vi "读取CODMn数据波形.vi"() -> ()   [LabVIEW 2016]
uses:
  System.Windows.Forms
  <vilib>/DataGrid for LabVIEW/source/GridColumn/ColumnDefinition.ctl
  <vilib>/DataGrid for LabVIEW/source/GridColumn/ColumnType.ctl
  <vilib>/Utility/miscctls.llb/LVPointTypeDef.ctl
  <vilib>/Waveform/WDTFileIO.llb/Read Waveform from File.vi
  <vilib>/DataGrid for LabVIEW/source/DataGridView/DataGridView.lvclass
  D:/Program Files (x86)/National Instruments/LabVIEW 2016/examples/DataGrid for LabVIEW/DataGrid.lvlib
  <vilib>/DataGrid for LabVIEW/source/Events/CellValueChanged/CellValueChanged.lvclass
  <vilib>/DataGrid for LabVIEW/source/Events/CellClick/CellClick.lvclass
  <vilib>/DataGrid for LabVIEW/source/Events/KeyDown/KeyDown.lvclass
  <vilib>/DataGrid for LabVIEW/source/GridColumn/GridColumn.lvclass
panel:
  in  "进度值":i32
  in  "当前温度曲线":bool
  out "下拉列表":u16(ring)
  in  "Discard?":bool
  in  "查询":bool
  in  "簇":cluster{"数据起始时间":timestamp, "数据终止时间":timestamp}
  in  "当前滴定曲线":bool
  in  "打开波形文件":bool
  in  "关闭":bool
  out "数组":T2(array[cluster]) {"MinWidth" min=2 step=1; "AutoSizeMode" items=["None"=1, "ColumnHeader"=2, "AllCellsExceptHeader"=4, "AllCells"=6, "DisplayedCellsExceptHeader"=8, "DisplayedCells"=10, "Fill"=16]; "FillWeight" min=1 max=100}
  out "Events":string
  in  "# of Rows":i32=15
  in  "ColumnSetup":T3[](array[typedef])=[{"name"="Text", "caption"="Text", "datatype"=enum."string", "Params"="", "AutoSizeMode"=2, "FillWeight"=10.0, "MinWidth"=25, "tooltip"="Text The quick brown fox jumps over the lazy dog"}, {"name"="Details", "caption"="Details", "datatype"=enum."string", "Params"="", "AutoSizeMode"=16, "FillWeight"=100.0, "MinWidth"=150, "tooltip"="Details The quick brown fox jumps over the lazy dog"}, {"name"="Time", "caption"="", "datatype"=enum."timestamp", "Params"="", "AutoSizeMode"=1, "FillWeight"=1.0, "MinWidth"=120, "tooltip"="Time The quick brown fox jumps over the lazy dog"}, {"name"="Selection", "caption"="", "datatype"=enum."combo", "Params"="One|Two|Three", "AutoSizeMode"=6, "FillWeight"=1.0, "MinWidth"=80, "tooltip"="Selection The quick brown fox jumps over the lazy dog"}, {"name"="Function", "caption"="", "datatype"=enum."button", "Params"="", "AutoSizeMode"=6, "FillWeight"=1.0, "MinWidth"=50, "tooltip"="Function The quick brown fox jumps over the lazy dog"}, {"name"="Value", "caption"="", "datatype"=enum."numeric", "Params"="", "AutoSizeMode"=6, "FillWeight"=1.0, "MinWidth"=10, "tooltip"="Value The quick brown fox jumps over the lazy dog"}, {"name"="Active", "caption"="", "datatype"=enum."check", "Params"="", "AutoSizeMode"=6, "FillWeight"=1.0, "MinWidth"=10, "tooltip"=""}, {"name"="Status", "caption"="", "datatype"=enum."image", "Params"="", "AutoSizeMode"=6, "FillWeight"=1.0, "MinWidth"=10, "tooltip"=""}, {"name"="Link", "caption"="", "datatype"=enum."link", "Params"="", "AutoSizeMode"=1, "FillWeight"=100.0, "MinWidth"=50, "tooltip"=""}] {"MinWidth" min=2 step=1; "AutoSizeMode" items=["None"=1, "ColumnHeader"=2, "AllCellsExceptHeader"=4, "AllCells"=6, "DisplayedCellsExceptHeader"=8, "DisplayedCells"=10, "Fill"=16]; "FillWeight" min=1 max=100}
  in  "DataGridView":refnum<k24>(container)
  # "加载中，请稍后......"
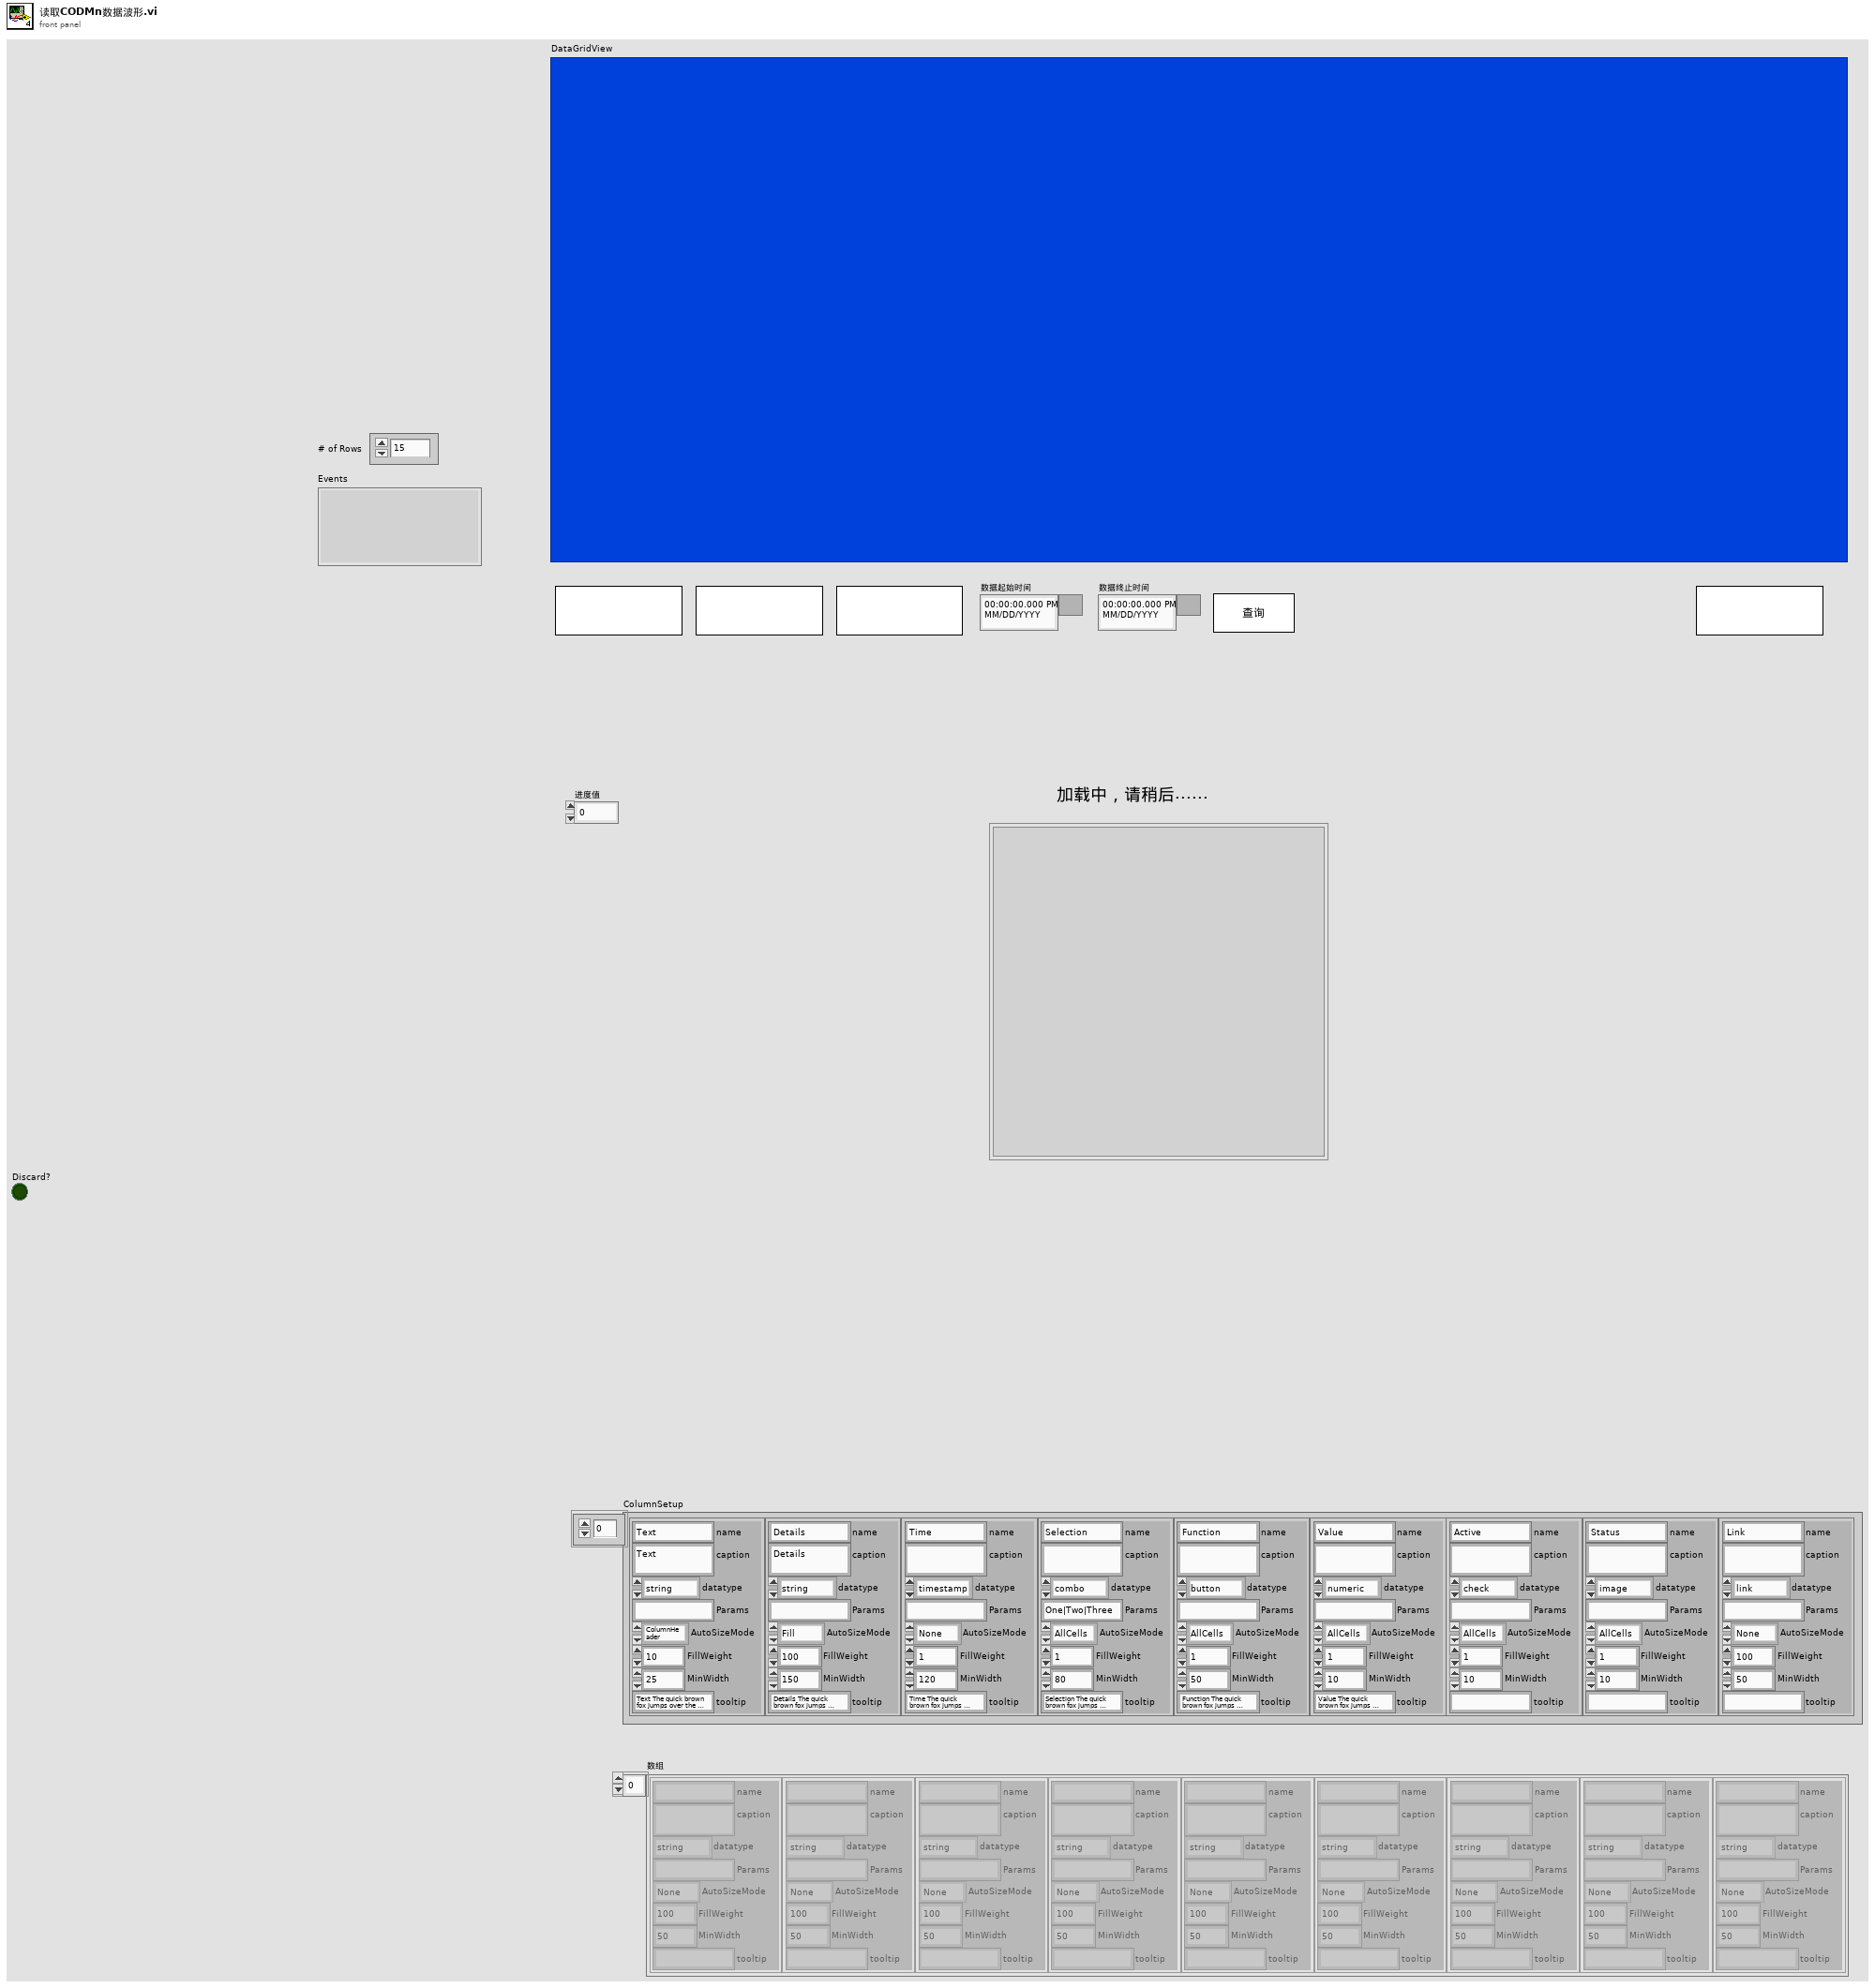
[diagram p1: front panel]
types:
  T1 = typedef "DataGrid.lvlib/GridColumn.lvclass/ColumnType.ctl" = enum16{"string", "image", "check", "numeric", "timestamp", "button", "combo", "link"}
  T2 = cluster{"name":string, "caption":string, "datatype":T1, "Params":string, "AutoSizeMode":i32, "FillWeight":sgl, "MinWidth":u32, "tooltip":string}[]
  T3 = typedef "DataGrid.lvlib/GridColumn.lvclass/ColumnDefinition.ctl" = cluster{"name":string, "caption":string, "datatype":T1, "Params":string, "AutoSizeMode":i32, "FillWeight":sgl, "MinWidth":u32, "tooltip":string}
  T4 = typedef "LVPointTypeDef.ctl" = cluster{"Horizontal":i16, "Vertical":i16}
  T5 = cluster{"Alt":bool, "Control":bool, "KeyCode":i32, "KeyData":i32, "KeyValue":i32, "Modifiers":i32, "Shift":bool}
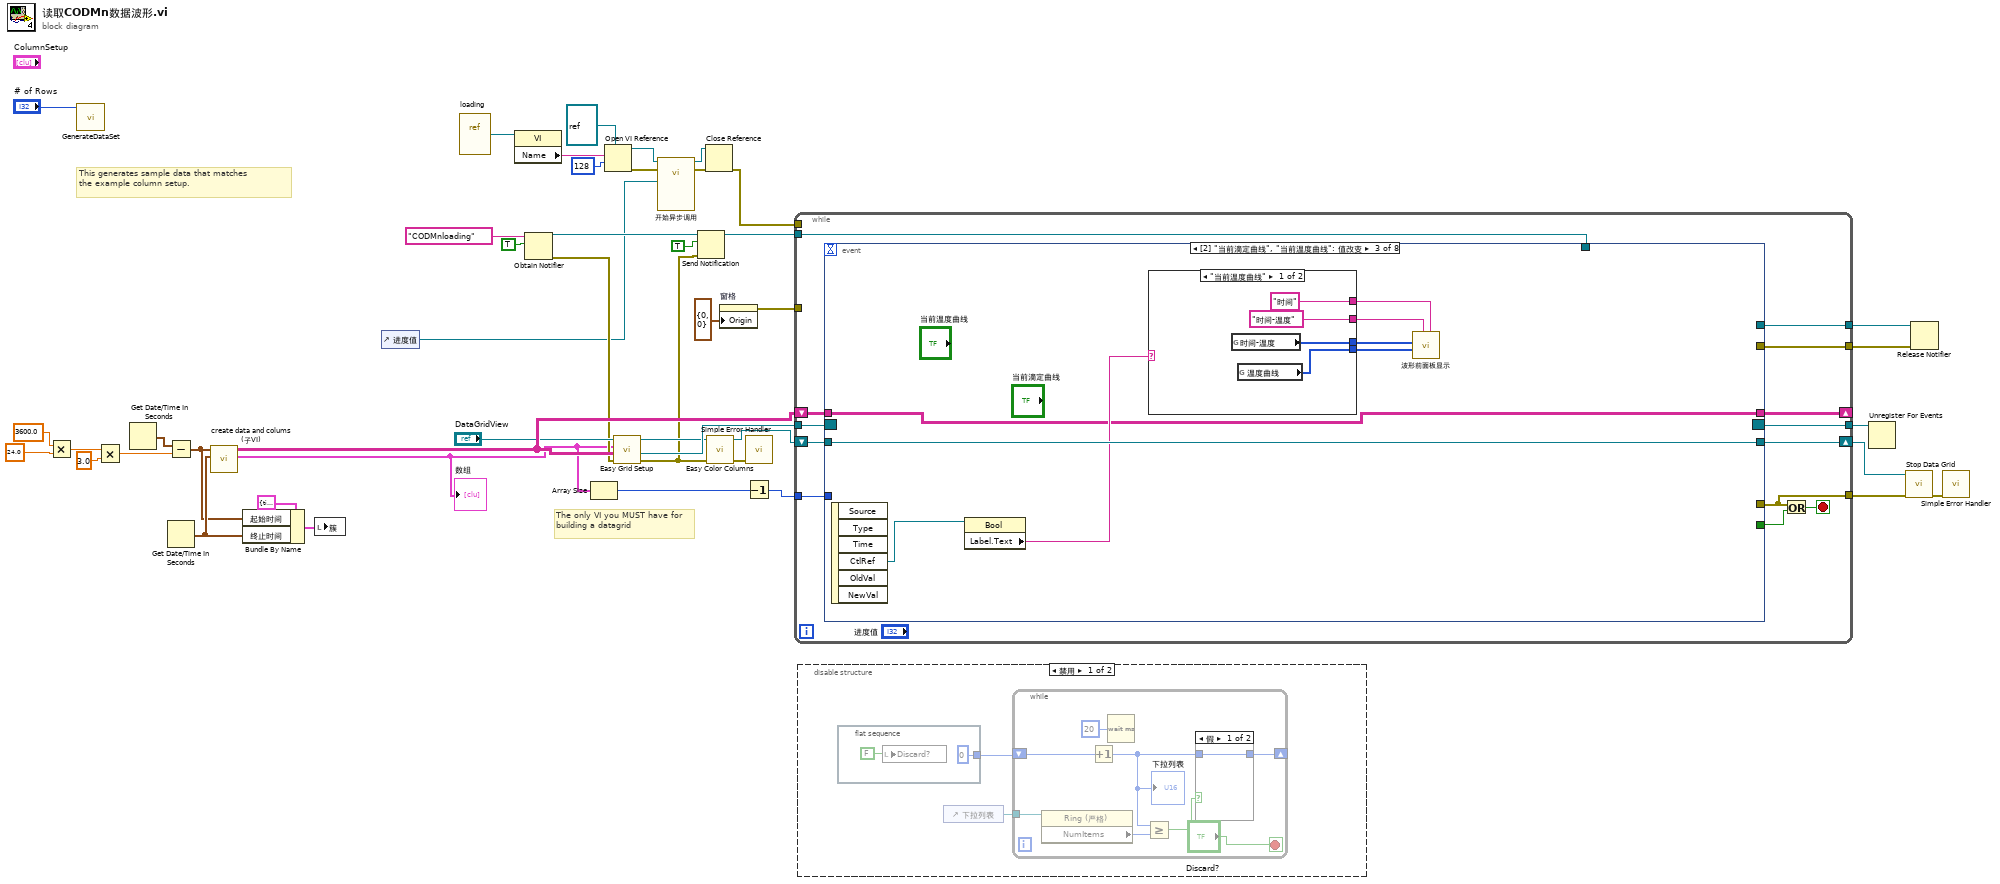
[diagram p0: block diagram]
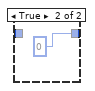
[diagram p2: hidden frame]
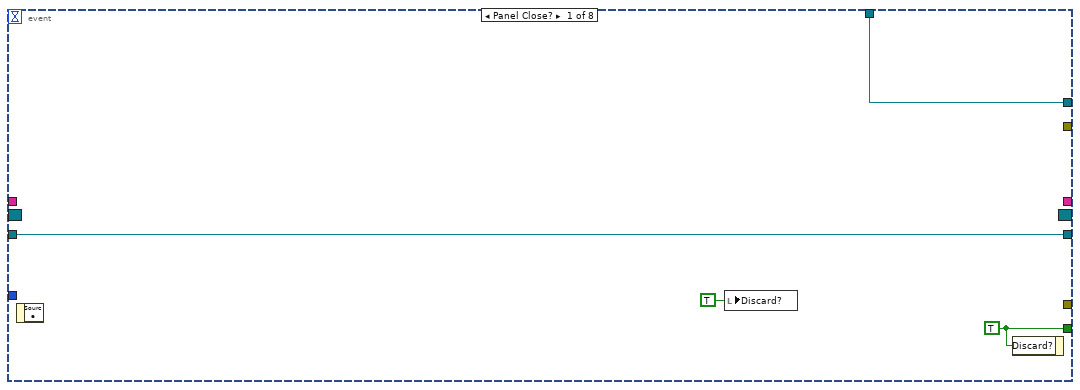
[diagram p4: hidden frame]
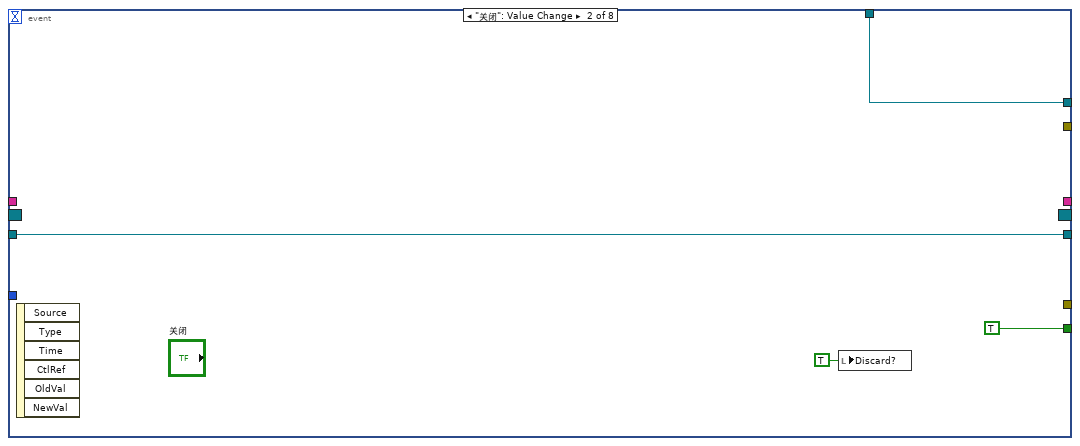
[diagram p5: hidden frame]
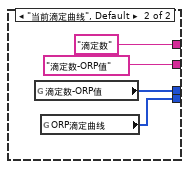
[diagram p6: hidden frame]
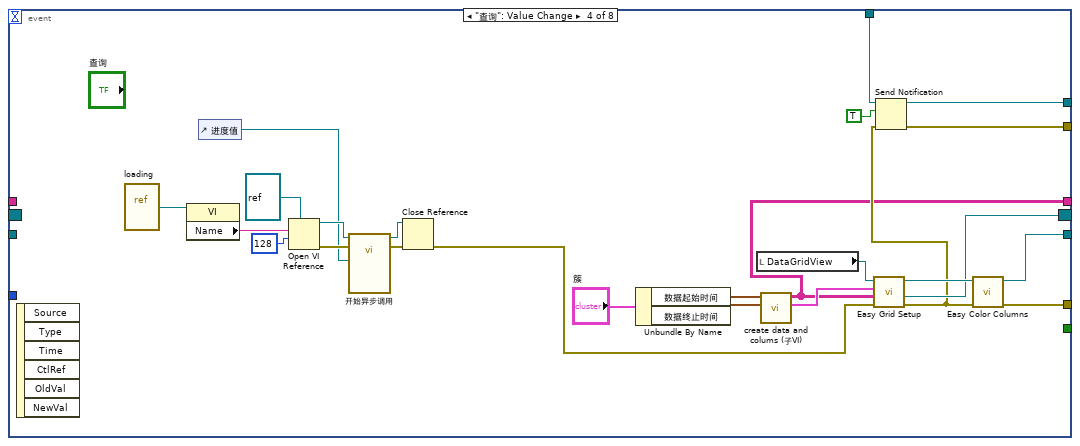
[diagram p7: hidden frame]
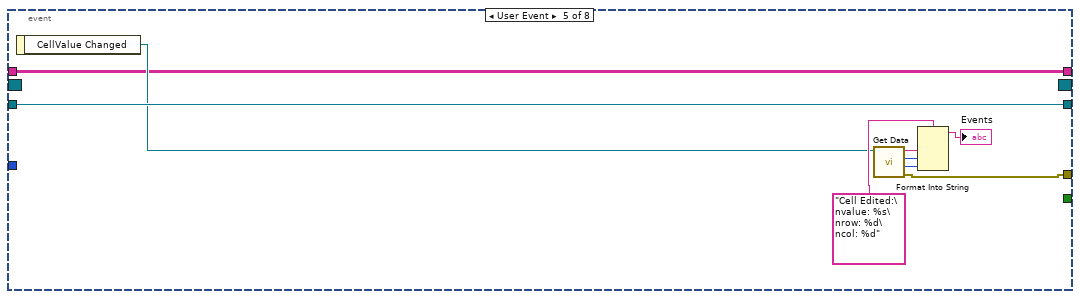
[diagram p8: hidden frame]
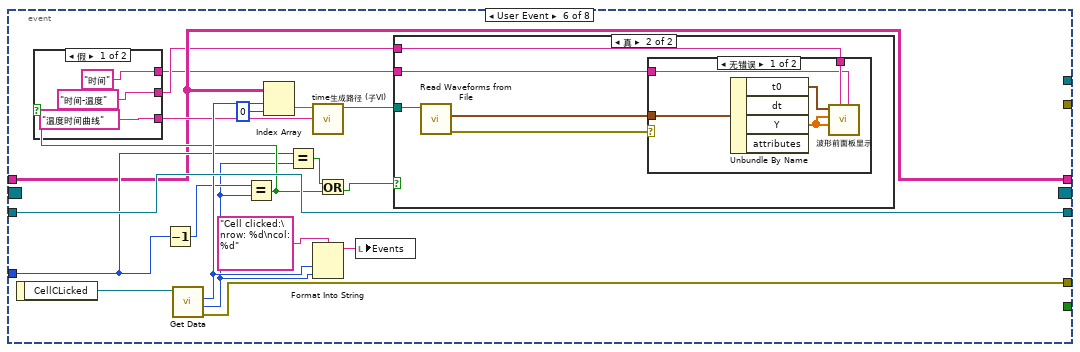
[diagram p9: hidden frame]
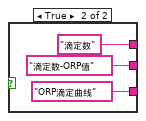
[diagram p10: hidden frame]
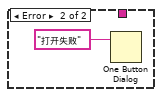
[diagram p12: hidden frame]
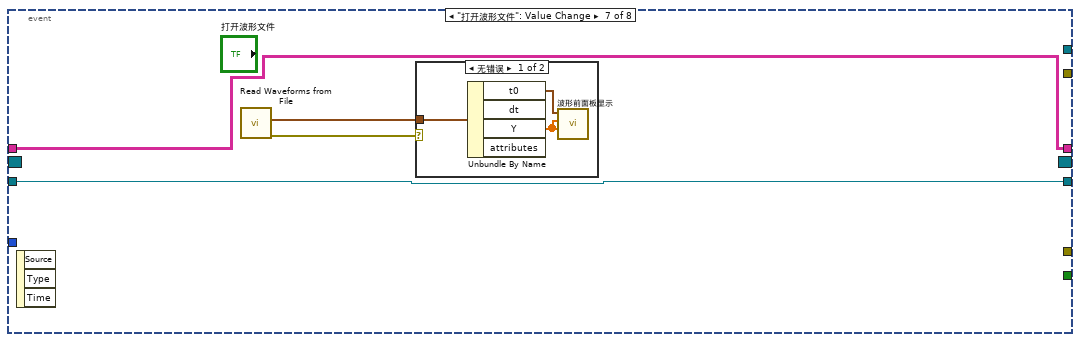
[diagram p13: hidden frame]
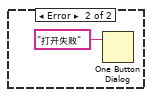
[diagram p14: hidden frame]
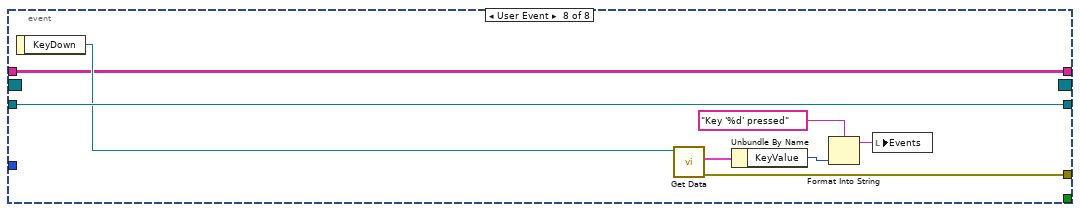
[diagram p15: hidden frame]
diagram:
  # "The only VI you MUST have for building a datagrid"
  # "This generates sample data that matches\nthe example column setup."
  n1 = Multiply(x=3600.0, y=24.0) -> (x*y=w32:dbl)
  n2 = call <vilib>:"GenerateDataSet.vi"("Records"="# of Rows") -> ()  [unwired: 10 in, 1 out]
  n3 = Multiply(x=w32, y=3.0) -> (x*y=w30:dbl)
  n4 = Get Date/Time In Seconds() -> (seconds since 1Jan1904=w35:timestamp)
  n5 = Subtract(x=w35, y=w30) -> (x-y=w25:timestamp)
  n6 = Get Date/Time In Seconds() -> (seconds since 1Jan1904=w26:timestamp)
  n7 = call "create data and colums (子VI).vi"("结束时间"=w26, "seconds since 1Jan1904"=w25) -> ("ColumnSetup"=w5:T2, "DataSource Data"=w36:string[][])  [unwired: 8 in]
  "数组" <- w5
  n8 = Bundle By Name(cluster=cluster{"起始时间":timestamp, "终止时间":timestamp} {"起始时间"=timestamp(0 s since 1904-01-01), "终止时间"=timestamp(0 s since 1904-01-01)} ("簇"), "起始时间"=w25, "终止时间"=w26) -> (w28:cluster{"起始时间":timestamp, "终止时间":timestamp})
  n9 = local write "簇"(w28) -> ()
  n10 = control-ref of="进度值"() -> (w1:refnum<vi>)
  n11 = vi-ref "loading.vi"() -> (w8:refnum<vi>)
  n12 = property class="VI"(reference=w8) -> ("Name"=w14:string)  [unwired: 1 in, 2 out]
  n13 = Obtain Notifier(name (unnamed)="CODMnloading" ("名称（未命名）"), notification data type=TRUE) -> (notifier out=w19:refnum<notifier>, error out=w18:errorcluster)  [unwired: 2 in, 1 out]
  n14 = Array Size(array=w5) -> (size(s)=w4:i32)
  n15 = Open VI Reference(type specifier VI Refnum (for type only)=refnum<vi> refnum, vi path=w14, options=128 ("选项")) -> (vi reference=w12:refnum<vi>, error out=w11:errorcluster)  [unwired: 3 in]
  n16 = call <vilib>:"Easy Grid Setup.vi"("error in"=w18, "DataSource Data"=w36, "ColumnSetup"=w5, "DataGridView"="DataGridView") -> ("error out"=w20:errorcluster, "registeredEvents"=w44:refnum<event-registration>, "DataGrid out"=w43:refnum<class "DataGridView.lvclass">)  [unwired: 4 in, 1 out]
  n17 = call-by-ref "开始异步调用"(reference=w12, error in=w11, "值"=w1) -> (reference out=w9:refnum<vi>, error out=w10:errorcluster)  [unwired: 10 in, 1 out]
  n18 = Send Notification(notification=TRUE ("通知"), notifier=w19, error in (no error)=w20) -> (notifier out=w17:refnum<notifier>)  [unwired: 1 out]
  n19 = Close Reference(reference=w9, error in (no error)=w10) -> (error out=w6:errorcluster)
  n20 = call <vilib>:"Easy Color Columns.vi"("error in (no error)"=w20, "DataGridView in"=w43) -> ("error out"=w40:errorcluster, "DataGridView out"=w42:refnum<class "DataGridView.lvclass">)  [unwired: 8 in]
  n21 = property on="窗格" class="Pane"("Origin"=T4 {"Horizontal"=0, "Vertical"=0} ("原点")) -> (error out=w2:errorcluster)  [unwired: 2 in, 1 out]
  n22 = call <vilib>:"Simple Error Handler.vi"("error in (no error)"=w40) -> ()  [unwired: 4 in, 5 out]
  n23 = Decrement(x=w4) -> (x-1=w24:i32)
  n24 = while {
    tunnel: w44 -> [w58]
    shift-right: [w56] -> w39
    shift-left: w42 -> [w57]
    tunnel: [w55] -> w41
    tunnel: [w53] -> w38
    tunnel: w24 -> [w50]
    tunnel: w17 -> [w49]
    tunnel: [w48] -> w16
    tunnel: [w47] -> w15
    tunnel: w6 -> [_]
    tunnel: w2 -> [_]
    shift-right: [w46] -> _
    shift-left: w36 -> [w51]
    stop <- w52 stop-if-true
    n25 = event shown="[2] \"当前滴定曲线\", \"当前温度曲线\": 值改变" {
      selector: w58 -> [_ _ _ _ _ _ _ _]
      dyn-events: [_ _ _ w105 _ _ _ _] -> w55
      timeout: _ -> [_ _ _ _ _ _ _ _]
      tunnel: [w62 TRUE ("Discard?") _ _ _ _ _ _] -> w54
      tunnel: w57 -> [w61 w66 w74 _ w114 w134 w156 w168]
      tunnel: [w61 w66 w74 w106 w114 w134 w156 w168] -> w56
      tunnel: [_ _ _ w99 w109 w131 _ w162] -> w53
      tunnel: w50 -> [_ _ _ _ _ w121 _ _]
      tunnel: w51 -> [_ _ w67 _ w108 w119 w153 w161]
      tunnel: w49 -> [w59 w63 _ w88 _ _ _ _]
      tunnel: [w59 w63 _ w86 _ _ _ _] -> w48
      tunnel: [_ _ _ w85 _ _ _ _] -> w47
      tunnel: [_ _ w67 w84 w108 w119 w153 w161] -> w46
      event Panel Close? {
        w62 = TRUE ("Discard?")
        n26 = event-data() -> ()  [unwired: 1 in, 1 out]
        n27 = local write "Discard?"(TRUE ("Discard?")) -> ()
        n28 = event-data("Discard?"=w62) -> ()  [unwired: 1 in, 1 out]
      }
      event "关闭": Value Change {
        n29 = event-data() -> ()  [unwired: 1 in, 6 out]
        n30 = local write "Discard?"(TRUE ("Discard?")) -> ()
      }
      event "当前滴定曲线", "当前温度曲线": Value Change {
        n31 = event-data() -> ("CtlRef"=w71:refnum<vi>)  [unwired: 1 in, 5 out]
        n32 = property class="Bool"(reference=w71) -> ("Label.Text"=w70:string)  [unwired: 1 in, 2 out]
        n33 = case shown="\"当前温度曲线\"" w70 {
          tunnel: [w77 w82] -> w73
          tunnel: [w78 w81] -> w72
          tunnel: ["时间-温度" ("标题.文本") "滴定数-ORP值" ("标题.文本")] -> w69
          tunnel: ["时间" ("X标尺.名称标签.文本") "滴定数" ("X标尺.名称标签.文本")] -> w68
          frame "当前温度曲线" {
            n34 = global read "VARCODMn全局变量.vi" "时间-温度"() -> (w78:u16[])
            n35 = global read "VARCODMn全局变量.vi" "温度曲线"() -> (w77:u16[])
          }
          frame "当前滴定曲线", Default {
            n36 = global read "VARCODMn全局变量.vi" "滴定数-ORP值"() -> (w81:u16[])
            n37 = global read "VARCODMn全局变量.vi" "ORP滴定曲线"() -> (w82:u16[])
          }
        }
        n38 = call "波形前面板显示.vi"("X标尺.名称标签.文本"=w68, "标题.文本"=w69, "ORP滴定曲线"=w73, "滴定数-ORP值"=w72) -> ()  [unwired: 8 in]
      }
      event "查询": Value Change {
        n39 = event-data() -> ()  [unwired: 1 in, 6 out]
        n40 = vi-ref "loading.vi"() -> (w92:refnum<vi>)
        n41 = property class="VI"(reference=w92) -> ("Name"=w98:string)  [unwired: 1 in, 2 out]
        n42 = control-ref of="进度值"() -> (w83:refnum<vi>)
        n43 = Open VI Reference(type specifier VI Refnum (for type only)=refnum<vi> refnum, vi path=w98, options=128 ("选项")) -> (vi reference=w96:refnum<vi>, error out=w95:errorcluster)  [unwired: 3 in]
        n44 = call-by-ref "开始异步调用"(reference=w96, error in=w95, "值"=w83) -> (reference out=w93:refnum<vi>, error out=w94:errorcluster)  [unwired: 10 in, 1 out]
        n45 = Close Reference(reference=w93, error in (no error)=w94) -> (error out=w90:errorcluster)
        n46 = Unbundle By Name("簇") -> ("数据起始时间"=w103:timestamp, "数据终止时间"=w102:timestamp)
        n47 = local read "DataGridView"() -> (w100:refnum<k24>)
        n48 = call "create data and colums (子VI).vi"("结束时间"=w102, "seconds since 1Jan1904"=w103) -> ("ColumnSetup"=w101:T2, "DataSource Data"=w84:string[][])  [unwired: 8 in]
        n49 = call <vilib>:"Easy Grid Setup.vi"("error in"=w90, "DataSource Data"=w84, "ColumnSetup"=w101, "DataGridView"=w100) -> ("error out"=w87:errorcluster, "registeredEvents"=w105:refnum<event-registration>, "DataGrid out"=w107:refnum<class "DataGridView.lvclass">)  [unwired: 4 in, 1 out]
        n50 = Send Notification(notification=TRUE ("通知"), notifier=w88, error in (no error)=w87) -> (notifier out=w86:refnum<notifier>, error out=w85:errorcluster)
        n51 = call <vilib>:"Easy Color Columns.vi"("error in (no error)"=w87, "DataGridView in"=w107) -> ("error out"=w99:errorcluster, "DataGridView out"=w106:refnum<class "DataGridView.lvclass">)  [unwired: 8 in]
      }
      event User Event {
        n52 = event-data() -> ("CellValue Changed"=w113:refnum<class "Abstract EVENT.lvclass">)  [unwired: 1 in]
        n53 = call <vilib>:"Get Data.vi"("DataGrid.lvlib:Abstract EVENT.lvclass"=w113) -> ("error out"=w109:errorcluster, "column"=w110:i32, "row"=w111:i32, "cell value"=w112:string)  [unwired: 7 in]
        n54 = Format Into String(format string="Cell Edited:\nvalue: %s\nrow: %d\ncol: %d" ("message"), w112, w111, w110) -> (resulting string=→"Events":string)  [unwired: 2 in, 1 out]
      }
      event User Event {
        n55 = event-data() -> ("CellCLicked"=w132:refnum<class "Abstract EVENT.lvclass">)  [unwired: 1 in]
        n56 = Decrement(x=w121) -> (x-1=w124:i32)
        n57 = call <vilib>:"Get Data.vi"("DataGrid.lvlib:Abstract EVENT.lvclass"=w132) -> ("error out"=w131:errorcluster, "column"=w122:i32, "row"=w129:i32)  [unwired: 8 in]
        n58 = Equal?(x=w124, y=w122) -> (x = y?=w123:bool)
        n59 = case shown="假" w123 {
          tunnel: ["温度时间曲线" ("名称或相对路径") "ORP滴定曲线" ("名称或相对路径")] -> w126
          tunnel: ["时间-温度" ("标题.文本") "滴定数-ORP值" ("标题.文本")] -> w118
          tunnel: ["时间" ("X标尺.名称标签.文本") "滴定数" ("X标尺.名称标签.文本")] -> w117
          frame False {
          }
          frame True {
          }
        }
        n60 = Index Array(array=w119, index (row)=w129, index (col)=0 ("禁用的索引 (列)")) -> (element=w128:string)
        n61 = Equal?(x=w121, y=w122) -> (x = y?=w120:bool)
        n62 = call "time生成路径 (子VI).vi"("名称或相对路径"=w126, "时间"=w128) -> ("appended path"=w127:path)  [unwired: 9 in]
        n63 = Format Into String(format string="Cell clicked:\nrow: %d\ncol: %d" ("message"), w129, w122) -> (resulting string=w135:string)  [unwired: 2 in, 1 out]
        n64 = Or(x=w120, y=w123) -> (x .or. y?=w125:bool)
        n65 = local write "Events"(w135) -> ()
        n66 = case shown="真" w125 {
          tunnel: w127 -> [_ w144]
          tunnel: w118 -> [_ w143]
          tunnel: w117 -> [_ w142]
          frame False {
          }
          frame True {
            n67 = call-poly <vilib>:"Read Waveforms from File.vi"("file path (dialog if empty)"=w144) -> ("error out"=w146:errorcluster, "first waveform in record"=w145:waveform(dbl))  [unwired: 5 in, 2 out]
            n68 = case shown="无错误" w146 {
              tunnel: w145 -> [w151 _]
              tunnel: w143 -> [w148 _]
              tunnel: w142 -> [w147 _]
              frame No Error {
                n69 = Unbundle By Name(w151) -> ("t0"=w150:timestamp, "Y"=w149:dbl[])  [unwired: 2 out]
                n70 = call "波形前面板显示.vi"("X标尺.名称标签.文本"=w147, "标题.文本"=w148, "ORP滴定曲线"=w149, "滴定数-ORP值"=w149, "波形时间"=w150) -> ()  [unwired: 7 in]
              }
              frame Error {
                n71 = One Button Dialog(message="打开失败" ("消息")) -> ()  [unwired: 1 in, 1 out]
              }
            }
          }
        }
      }
      event "打开波形文件": Value Change {
        n72 = event-data() -> ()  [unwired: 1 in, 3 out]
        n73 = call-poly <vilib>:"Read Waveforms from File.vi"() -> ("error out"=w155:errorcluster, "first waveform in record"=w154:waveform(dbl))  [unwired: 6 in, 2 out]
        n74 = case shown="无错误" w155 {
          tunnel: w154 -> [w159 _]
          frame No Error {
            n75 = Unbundle By Name(w159) -> ("t0"=w158:timestamp, "Y"=w157:dbl[])  [unwired: 2 out]
            n76 = call "波形前面板显示.vi"("ORP滴定曲线"=w157, "滴定数-ORP值"=w157, "波形时间"=w158) -> ()  [unwired: 9 in]
          }
          frame Error {
            n77 = One Button Dialog(message="打开失败" ("消息")) -> ()  [unwired: 1 in, 1 out]
          }
        }
      }
      event User Event {
        n78 = event-data() -> ("KeyDown"=w167:refnum<class "Abstract EVENT.lvclass">)  [unwired: 1 in]
        n79 = call <vilib>:"Get Data.vi"("DataGrid.lvlib:Abstract EVENT.lvclass"=w167) -> ("error out"=w162:errorcluster, "output cluster"=w164:T5)  [unwired: 9 in]
        n80 = Unbundle By Name(w164) -> ("KeyValue"=w163:i32)
        n81 = Format Into String(format string="Key '%d' pressed" ("message"), w163) -> (resulting string=w166:string)  [unwired: 2 in, 1 out]
        n82 = local write "Events"(w166) -> ()
      }
    }
    n83 = Or(x=w53, y=w54) -> (x .or. y?=w52:bool)
  }
  n84 = disable-structure shown="禁用" {
    frame Disabled {
      n85 = flat-sequence {
        tunnel: [u16 0] -> w169
        frame #0 {
          n86 = local write "Discard?"(FALSE ("Discard?")) -> ()
        }
      }
      n87 = control-ref of="下拉列表"() -> (w170:refnum<vi>)
      n88 = while {
        shift-right: [w177] -> _
        shift-left: w169 -> [w180]
        tunnel: w170 -> [w179]
        stop <- "Discard?" stop-if-true
        n89 = property class="Ring (严格)"(reference=w179) -> ("NumItems"=w178:u32)  [unwired: 1 in, 2 out]
        n90 = Increment(x=w180) -> (x+1=w175:u16)
        "下拉列表" <- w175
        n91 = Wait (ms)(milliseconds to wait=u32 20 ("等待时间（毫秒）")) -> ()  [unwired: 1 out]
        n92 = Greater Or Equal?(x=w175, y=w178) -> (x >= y?=w176:bool)
        n93 = case shown="假" w176 {
          tunnel: [w181 u16 0] -> w177
          tunnel: w175 -> [w181 _]
          frame False {
          }
          frame True {
          }
        }
      }
    }
    frame Enabled {
    }
  }
  n94 = Unregister For Events(event registration refnum=w41) -> ()  [unwired: 1 in, 1 out]
  n95 = call <vilib>:"Stop Data Grid.vi"("error in (no error)"=w38, "DataGridView in"=w39) -> ("error out"=w37:errorcluster)  [unwired: 8 in, 1 out]
  n96 = Release Notifier(notifier=w16, error in (no error)=w15) -> ()  [unwired: 1 in, 3 out]
  n97 = call <vilib>:"Simple Error Handler.vi"("error in (no error)"=w37) -> ()  [unwired: 4 in, 5 out]
